vi "subSet2TierRebuildFlag.vi"(8 "error in (no error)":errorcluster, 11 "SolutionBuilder in":refnum<class "SolutionBuilder.lvclass">) -> (0 "error out":errorcluster, 3 "SolutionBuilder out":refnum<class "SolutionBuilder.lvclass">)   [LabVIEW 2019, in "SolutionBuilder.lvlib" / "SolutionBuilder.lvclass"]
uses:
  SolutionBuilder.lvclass
  SolutionBuilder.lvclass/SolutionBuilder.ctl
  ProjectItem/ProjectItem.lvclass
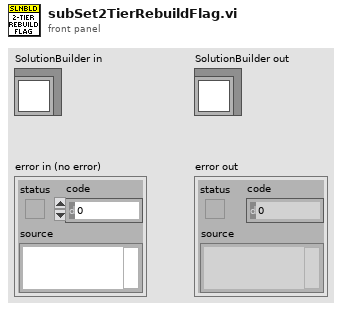
[diagram p1: front panel]
types:
  T1 = typedef "SolutionBuilder.lvlib/SolutionBuilder.lvclass/ProjectItemMap.ctl" = map{path, refnum<class "ProjectItem.lvclass">[]}
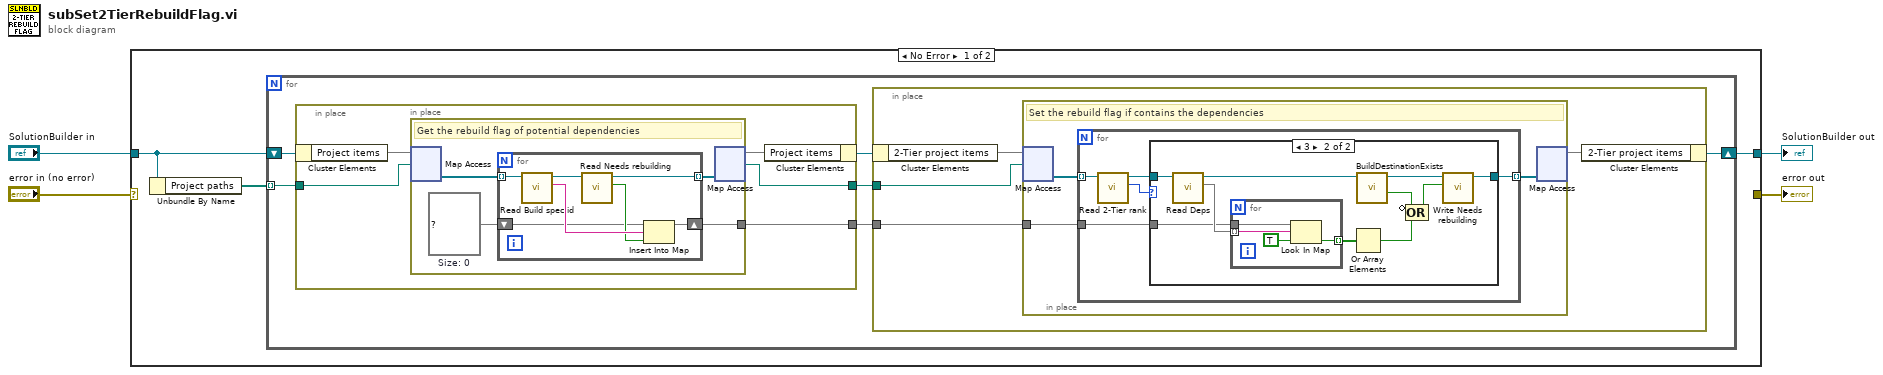
[diagram p0: block diagram]
diagram:
  n1 = case shown="No Error" "error in (no error)" {
    selector: "error in (no error)" -> [_ w58]
    tunnel: [_ w58] -> w3
    tunnel: [w6 w57] -> w1
    tunnel: "SolutionBuilder in" -> [w7 w57]
    frame No Error {
      n2 = Unbundle By Name(w7) -> ("Project paths"=w5:path[])
      n3 = for {
        shift-right: [w8] -> w6
        shift-left: w7 -> [w13]
        tunnel: w5 -> [w12] mode=indexing
        n4 = in-place {
          in-place-border: w12 -> [w44]
          in-place-border: [w42] -> w9
          in-place-border: [w41] -> w10
          n5 = in-place-cluster #1(w13) -> ("Project items"=w45:T1)
          n6 = in-place {
            in-place-border: [w46] -> w42
            w47 = map{string, bool} {}  # Size: 0
            # "Get the rebuild flag of potential dependencies"
            n7 = in-place-map #2(w45, w44) -> (w49:refnum<class "ProjectItem.lvclass">[])  [unwired: 1 in, 1 out]
            n8 = for {
              tunnel: w49 -> [w56] mode=indexing
              tunnel: [w54] -> w48 mode=indexing
              shift-right: [w51] -> w46
              shift-left: w47 -> [w50]
              n9 = call-dynamic "Read Build spec id.vi"("ProjectItem in"=w56) -> ("Build spec id"=w53:string, "ProjectItem out"=w55:refnum<class "ProjectItem.lvclass">)  [unwired: 9 in]
              n10 = call "Read Needs rebuilding.vi"("ProjectItem in"=w55) -> ("Needs rebuilding"=w52:bool, "ProjectItem out"=w54:refnum<class "ProjectItem.lvclass">)  [unwired: 9 in]
              n11 = Insert Into Map(map in=w50, key=w53, value=w52) -> (map out=w51:map{string, bool})  [unwired: 2 out]
            }
            n12 = in-place-map #2(w48) -> (w43:T1, w41:path)  [unwired: 1 in, 1 out]
          }
          n13 = in-place-cluster #1("Project items"=w43) -> (w11:refnum<class "SolutionBuilder.lvclass">)
        }
        n14 = in-place {
          in-place-border: w10 -> [w16]
          in-place-border: w9 -> [w14]
          n15 = in-place-cluster #3(w11) -> ("2-Tier project items"=w17:T1)
          n16 = in-place {
            in-place-border: w14 -> [w18]
            # "Set the rebuild flag if contains the dependencies"
            n17 = in-place-map #4(w17, w16) -> (w20:refnum<class "ProjectItem.lvclass">[])  [unwired: 1 in, 1 out]
            n18 = for {
              tunnel: w20 -> [w24] mode=indexing
              tunnel: [w25] -> w19 mode=indexing
              tunnel: w18 -> [w21]
              n19 = call "Read 2-Tier rank.vi"("ProjectItem in"=w24) -> ("2-Tier rank"=w22:u8, "ProjectItem out"=w23:refnum<class "ProjectItem.lvclass">)  [unwired: 9 in]
              n20 = case shown="3" w22 {
                tunnel: [w26 w33] -> w25
                tunnel: w23 -> [w26 w27]
                tunnel: w21 -> [_ w35]
                frame Default {
                }
                frame 3 {
                  n21 = call "Read Deps.vi"("ProjectItem in"=w27) -> ("Deps"=w36:set{string}, "ProjectItem out"=w32:refnum<class "ProjectItem.lvclass">)  [unwired: 9 in]
                  n22 = for {
                    tunnel: w36 -> [w40] mode=indexing
                    tunnel: [w38] -> w34 mode=indexing
                    tunnel: w35 -> [w37]
                    n23 = Look In Map(map=w37, key=w40, default value=TRUE) -> (value=w38:bool)  [unwired: 1 out]
                  }
                  n24 = Or Array Elements(Boolean array=w34) -> (logical OR=w29:bool)
                  n25 = call "BuildDestinationExists.vi"("ProjectItem in"=w32) -> ("Exists"=w30:bool, "ProjectItem out"=w31:refnum<class "ProjectItem.lvclass">)  [unwired: 7 in, 2 out]
                  n26 = Compound Arithmetic op=OR(invert w30, w29) -> (w28:bool)
                  n27 = call "Write Needs rebuilding.vi"("Needs rebuilding"=w28, "ProjectItem in"=w31) -> ("ProjectItem out"=w33:refnum<class "ProjectItem.lvclass">)  [unwired: 9 in]
                }
              }
            }
            n28 = in-place-map #4(w19) -> (w15:T1)  [unwired: 1 in, 2 out]
          }
          n29 = in-place-cluster #3("2-Tier project items"=w15) -> (w8:refnum<class "SolutionBuilder.lvclass">)
        }
      }
    }
    frame Error {
    }
  }
  "error out" <- w3
  "SolutionBuilder out" <- w1
